vi "ZStackDisplay.vi"() -> ()   [LabVIEW 2017]
panel:
  in  "LUT":cluster{i16, i16}(slide)={0, 4095} scale=0.0..4095.0
  in  "Image 1 Palette":enum16{""}(ring)
  in  "Image 1 Channel":enum16{""}(ring)
  out "Image 1":T1(plugin-control)
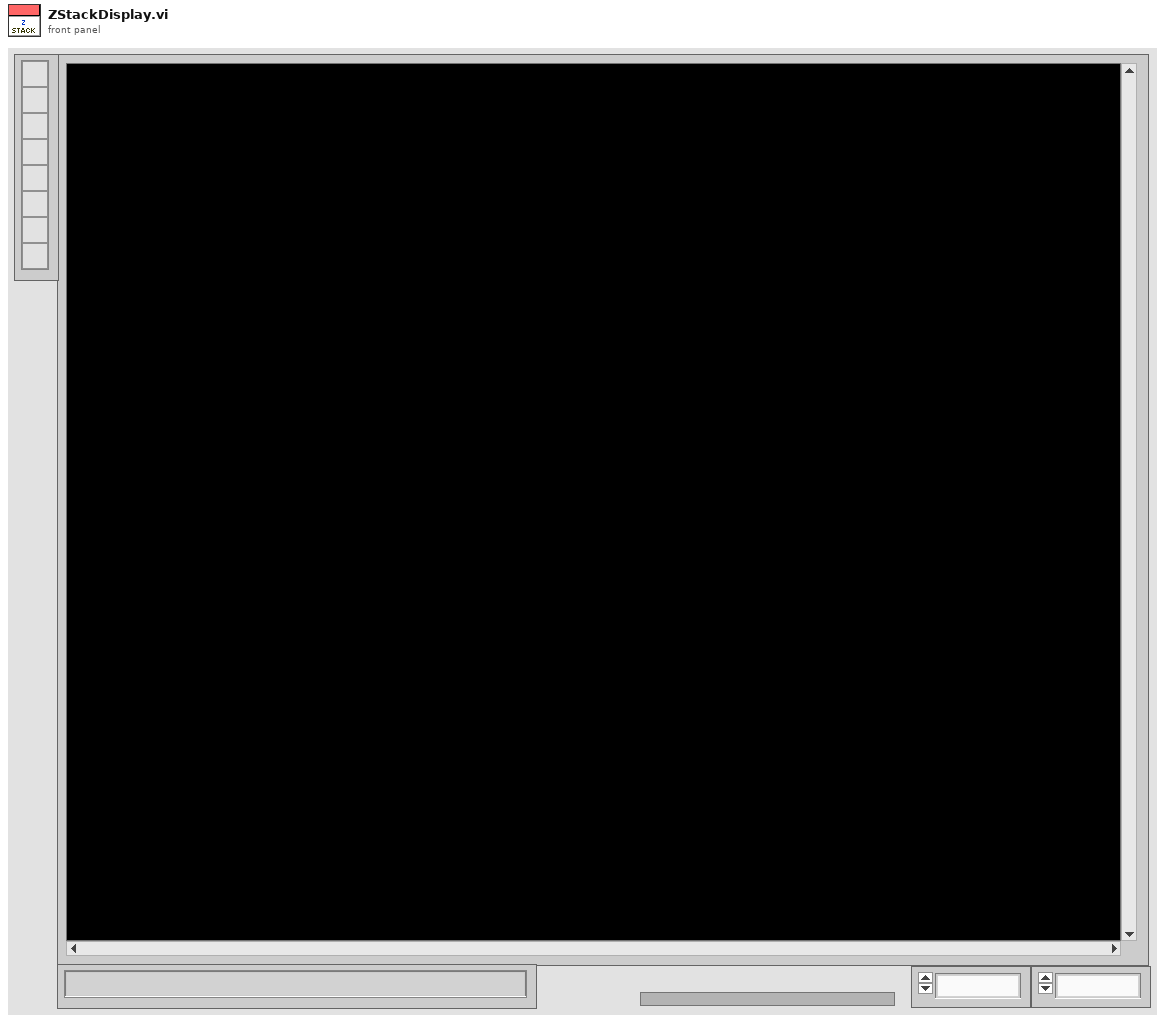
[diagram p1: front panel]
types:
  T1 = typedef "IMAQ Image.ctl" = refnum<image>
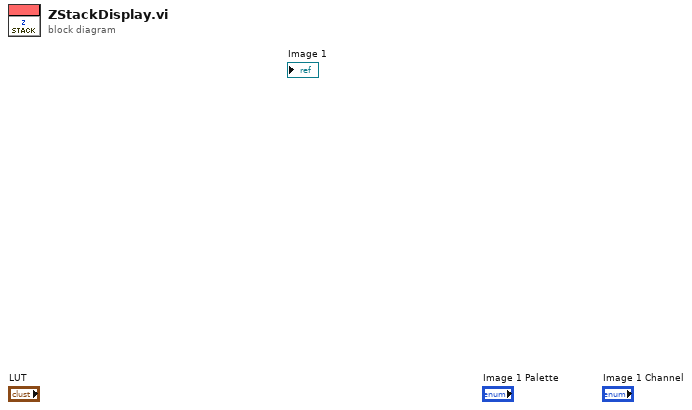
[diagram p0: block diagram]
diagram:
